vi "Control Matrix Sizing (SubVI).vi"(0 "Phase":dbl[](array[numeric]), 1 "Loops":dbl[](array[numeric]), 4 "Fire/Startup":dbl[](array[numeric]), 6 "Abort State":dbl[](array[numeric]), 7 "GO States":dbl[](array[numeric]), 8 "Sequences":dbl[](array[numeric]), 9 "Timer":dbl[](array[numeric]), 10 "Input Matrix":dbl[][](array[numeric]), 11 "Valve States":dbl[](array[numeric])) -> (3 "Output Matrix":dbl[][](array[numeric]))   [LabVIEW 2019]
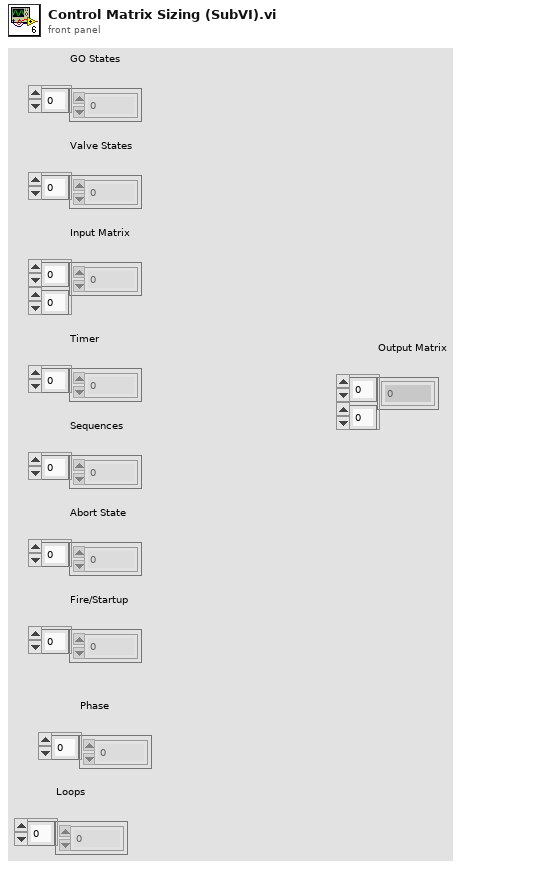
[diagram p1: front panel]
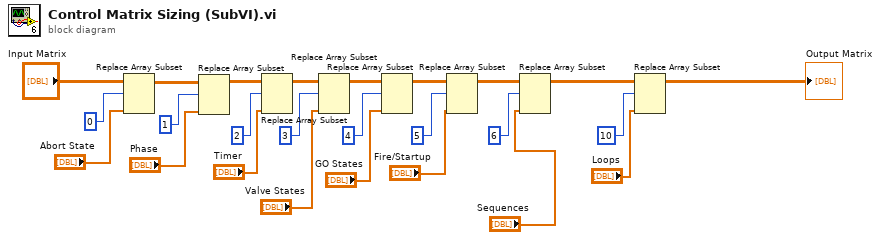
[diagram p0: block diagram]
diagram:
  n1 = Replace Array Subset(array="Input Matrix", new element="Abort State", index (row)=0) -> (w7:dbl[][])  [unwired: 1 in]
  n2 = Replace Array Subset(array=w7, new element="Phase", index (row)=1) -> (w1:dbl[][])  [unwired: 1 in]
  n3 = Replace Array Subset(array=w1, new element="Timer", index (row)=2) -> (w12:dbl[][])  [unwired: 1 in]
  n4 = Replace Array Subset(array=w12, new element="Valve States", index (row)=3) -> (w11:dbl[][])  [unwired: 1 in]
  n5 = Replace Array Subset(array=w11, new element="GO States", index (row)=4) -> (w10:dbl[][])  [unwired: 1 in]
  n6 = Replace Array Subset(array=w10, new element="Fire/Startup", index (row)=5) -> (w20:dbl[][])  [unwired: 1 in]
  n7 = Replace Array Subset(array=w20, new element="Sequences", index (row)=6) -> (w4:dbl[][])  [unwired: 1 in]
  n8 = Replace Array Subset(array=w4, new element="Loops", index (row)=10) -> (→"Output Matrix":dbl[][])  [unwired: 1 in]
